vi "Out_S2F35.vi"(8 "error in (no error)":errorcluster, 10 "S2F35":T1, 11 "S2 Message Class in":refnum<class "S2 Message Class.lvclass">) -> (0 "error out":errorcluster, 3 "S2 Message Class out":refnum<class "S2 Message Class.lvclass">)   [LabVIEW 2020, in "SECS Communication.lvlib" / "S2 Message Class.lvclass"]
uses:
  S2 Message Class.lvclass
  D:/Dropbox/SECS/SECS_GEM v1.0.7/Com/SECS Communication/SECS-II Class/SECS-II Class.lvclass
  S2F35.ctl
  SECS-II Class/Data Message_List.vi
  SECS-II Class/Data Message_U4.vi
  SECS-II Class/SECS-II Class.lvclass
  D:/Dropbox/SECS/SECS_GEM v1.0.7/Com/SECS Communication/S2 Message Class/S2 Message Class.lvclass
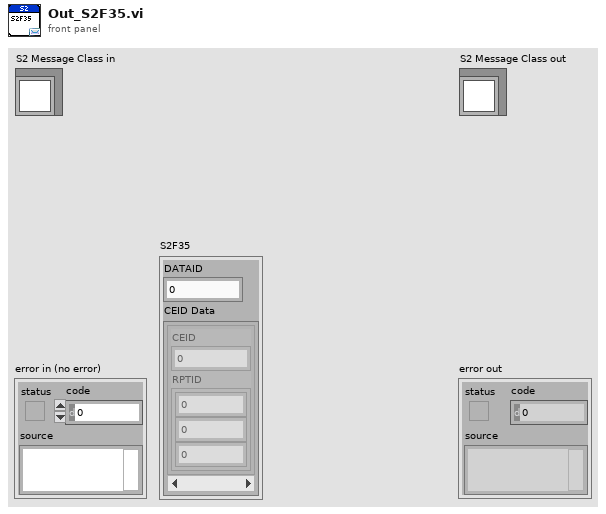
[diagram p1: front panel]
types:
  T1 = typedef "SECS Communication.lvlib/S2 Message Class.lvclass/S2F35.ctl" = cluster{"DATAID":u32, "CEID Data":cluster{"CEID":u32, "RPTID":u32[]}[]}
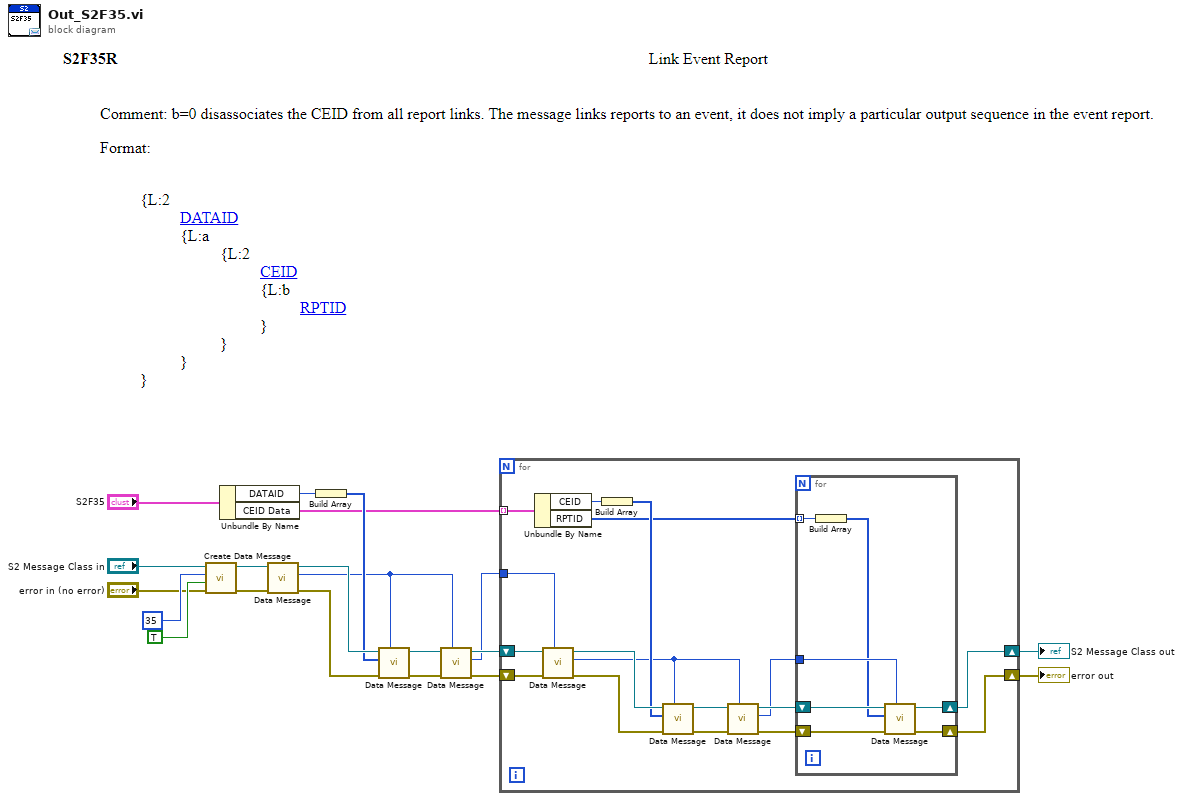
[diagram p0: block diagram]
diagram:
  n1 = call "Create Data Message.vi"("error in (no error)"="error in (no error)", "W-Bit"=TRUE, "Function"=u8 35, "SECS-II Class in"="S2 Message Class in") -> ("error out"=w16:errorcluster, "SECS-II Class out"=w15:refnum<class "S2 Message Class.lvclass">)  [unwired: 6 in]
  n2 = Unbundle By Name("S2F35") -> ("DATAID"=w11:u32, "CEID Data"=w3:cluster{"CEID":u32, "RPTID":u32[]}[])
  n3 = call-poly "Data Message.vi"("error in"=w16, "SECS-II Class in"=w15) -> ("error out"=w14:errorcluster, "Index"=w7:i32, "SECS-II Class out"=w13:refnum<class "S2 Message Class.lvclass">)  [unwired: 7 in]
  n4 = Build Array(w11) -> (w10:u32[])
  n5 = call-poly "Data Message.vi"("Parent Index"=w7, "error in"=w14, "Data"=w10, "SECS-II Class in"=w13) -> ("error out"=w9:errorcluster, "SECS-II Class out"=w8:refnum<class "S2 Message Class.lvclass">)  [unwired: 6 in]
  n6 = call-poly "Data Message.vi"("Parent Index"=w7, "error in"=w9, "SECS-II Class in"=w8) -> ("error out"=w6:errorcluster, "Index"=w4:i32, "SECS-II Class out"=w5:refnum<class "S2 Message Class.lvclass">)  [unwired: 6 in]
  n7 = for {
    shift-right: [w21] -> w1
    shift-left: w6 -> [w37]
    shift-right: [w22] -> w2
    shift-left: w5 -> [w36]
    tunnel: w4 -> [w28]
    tunnel: w3 -> [w33] mode=indexing
    n8 = Unbundle By Name(w33) -> ("CEID"=w32:u32, "RPTID"=w23:u32[])
    n9 = call-poly "Data Message.vi"("Parent Index"=w28, "error in"=w37, "SECS-II Class in"=w36) -> ("error out"=w35:errorcluster, "Index"=w27:i32, "SECS-II Class out"=w34:refnum<class "S2 Message Class.lvclass">)  [unwired: 6 in]
    n10 = Build Array(w32) -> (w31:u32[])
    n11 = call-poly "Data Message.vi"("Parent Index"=w27, "error in"=w35, "Data"=w31, "SECS-II Class in"=w34) -> ("error out"=w30:errorcluster, "SECS-II Class out"=w29:refnum<class "S2 Message Class.lvclass">)  [unwired: 6 in]
    n12 = call-poly "Data Message.vi"("Parent Index"=w27, "error in"=w30, "SECS-II Class in"=w29) -> ("error out"=w26:errorcluster, "Index"=w24:i32, "SECS-II Class out"=w25:refnum<class "S2 Message Class.lvclass">)  [unwired: 6 in]
    n13 = for {
      shift-right: [w39] -> w22
      shift-left: w25 -> [w44]
      shift-right: [w38] -> w21
      shift-left: w26 -> [w43]
      tunnel: w24 -> [w42]
      tunnel: w23 -> [w41] mode=indexing
      n14 = Build Array(w41) -> (w40:u32[])
      n15 = call-poly "Data Message.vi"("Parent Index"=w42, "error in"=w43, "Data"=w40, "SECS-II Class in"=w44) -> ("error out"=w38:errorcluster, "SECS-II Class out"=w39:refnum<class "S2 Message Class.lvclass">)  [unwired: 6 in]
    }
  }
  "error out" <- w1
  "S2 Message Class out" <- w2
